vi "Call gRPC Scripting.vi"(8 "error in":errorcluster, 9 "gRPC Service Name":string, 10 "proto File Path":path, 11 "PluginGenerator_MetaDataObj":refnum<class "PluginGenerator_MetaDataObj.lvclass">) -> (0 "error out":errorcluster, 3 "PluginGenerator_MetaDataObj out":refnum<class "PluginGenerator_MetaDataObj.lvclass">)   [LabVIEW 2021, in "Plugin Generator.lvlib"]
uses:
  Plugin Generator.lvlib
  PluginGenerator_MetaDataObj/PluginGenerator_MetaDataObj.lvclass
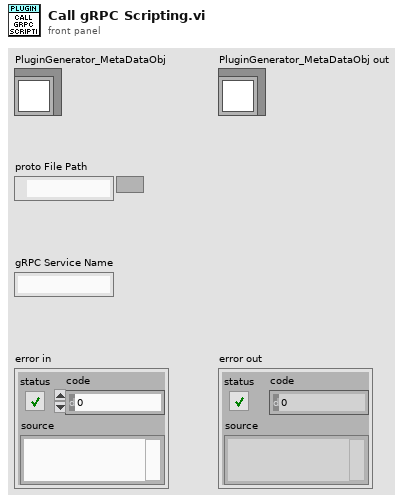
[diagram p1: front panel]
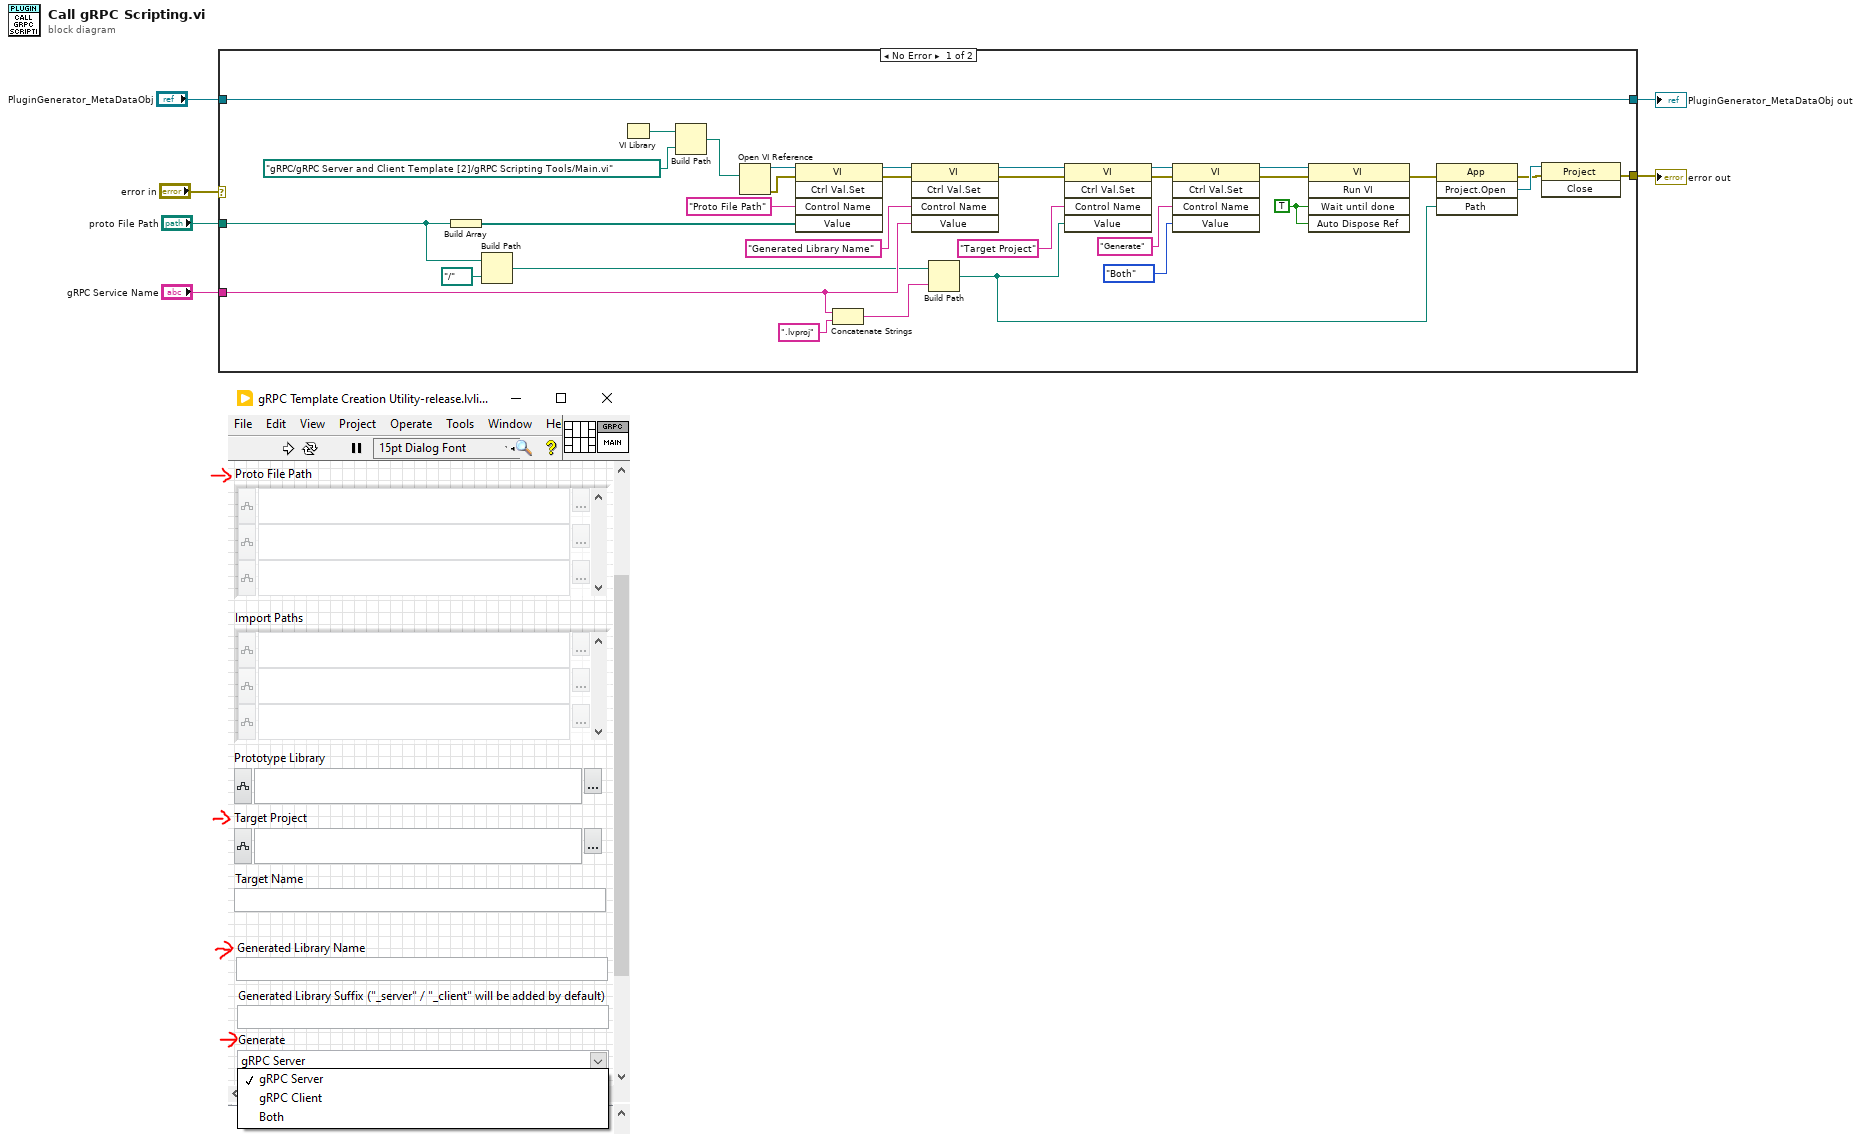
[diagram p0: block diagram]
diagram:
  n1 = case shown="No Error" "error in" {
    selector: "error in" -> [_ w40]
    tunnel: [w15 w40] -> w6
    tunnel: "gRPC Service Name" -> [w12 _]
    tunnel: "proto File Path" -> [w11 _]
    tunnel: [w7 w39] -> w2
    tunnel: "PluginGenerator_MetaDataObj" -> [w7 w39]
    frame No Error {
      w13 = TRUE ("Wait Until Done")
      n2 = Build Array(w11) -> (w20:path[])
      n3 = Build Path(base path=w11, name or relative path=path "../..") -> (appended path=w10:path)
      n4 = VI Library() -> (path=w38:path)
      n5 = Build Path(base path=w38, name or relative path=path "gRPC/gRPC Server and Client Template [2]/gRPC Scripting Tools/Main.vi") -> (appended path=w36:path)
      n6 = Open VI Reference(vi path=w36) -> (vi reference=w22:refnum<vi>, error out=w21:errorcluster)  [unwired: 5 in]
      n7 = invoke class="VI" method="Ctrl Val.Set"(reference=w22, error in=w21, "Control Name"="Proto File Path", "Value"=w20) -> (reference out=w34:refnum<vi>, error out=w33:errorcluster)  [unwired: 1 in, 3 out]
      n8 = Concatenate Strings(w12, ".lvproj" ("string")) -> (w18:string)
      n9 = invoke class="VI" method="Ctrl Val.Set"(reference=w34, error in=w33, "Control Name"="Generated Library Name", "Value"=w12) -> (reference out=w31:refnum<vi>, error out=w30:errorcluster)  [unwired: 1 in, 3 out]
      n10 = Build Path(base path=w10, name or relative path=w18) -> (appended path=w8:path)
      n11 = invoke class="VI" method="Ctrl Val.Set"(reference=w31, error in=w30, "Control Name"="Target Project", "Value"=w8) -> (reference out=w28:refnum<vi>, error out=w27:errorcluster)  [unwired: 1 in, 3 out]
      n12 = invoke class="VI" method="Ctrl Val.Set"(reference=w28, error in=w27, "Control Name"="Generate", "Value"=enum16{"gRPC Server", "gRPC Client", "Both"}."Both" ("Generate")) -> (reference out=w24:refnum<vi>, error out=w23:errorcluster)  [unwired: 1 in, 3 out]
      n13 = invoke class="VI" method="Run VI"(reference=w24, error in=w23, "Wait until done"=w13, "Auto Dispose Ref"=w13) -> (error out=w14:errorcluster)  [unwired: 1 in, 4 out]
      n14 = invoke class="App" method="Project.Open"(error in=w14, "Path"=w8) -> (error out=w16:errorcluster, "Project:Open"=w17:refnum<vi>)  [unwired: 2 in, 2 out]
      n15 = invoke class="Project" method="Close"(reference=w17, error in=w16) -> (error out=w15:errorcluster)  [unwired: 1 in, 2 out]
    }
    frame Error {
    }
  }
  "error out" <- w6
  "PluginGenerator_MetaDataObj out" <- w2
